vi "Memory.Pointer.Read.All.In Place.Safe (1D U8).vi"(8 "error in (no error)":errorcluster, 10 "buffer in":u8[](array[numeric]) format="%02x", 11 "Pointer in":refnum<class "Memory.Pointer.lvclass">) -> (0 "error out":errorcluster, 2 "buffer out":u8[](array[numeric]) format="%02x", 3 "Pointer out":refnum<class "Memory.Pointer.lvclass">)   [LabVIEW 2016, in "LabVIEW Memory Manager.lvlib" / "Memory.Pointer.lvclass"]
uses:
  Memory.Pointer.lvclass
  Memory.Pointer.lvclass/Memory.Pointer.ctl
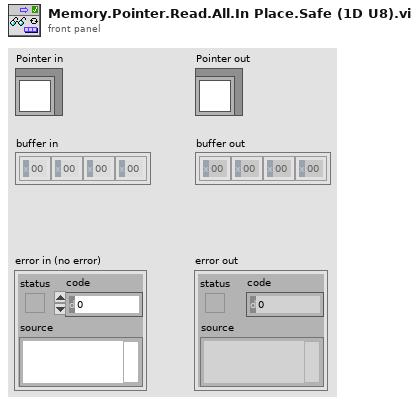
[diagram p1: front panel]
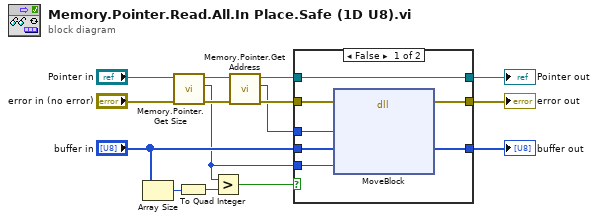
[diagram p0: block diagram]
diagram:
  n1 = Array Size(array="buffer in") -> (size(s)=w6:i32)
  n2 = call "Memory.Pointer.Get Size.vi"("error in (no error)"="error in (no error)", "Pointer in"="Pointer in") -> ("error out"=w15:errorcluster, "size"=w4:i64, "Pointer out"=w14:refnum<class "Memory.Pointer.lvclass">)  [unwired: 7 in]
  n3 = To Quad Integer(1:w6) -> (0:w5:i64)
  n4 = Greater?(x=w4, y=w5) -> (0:w1:bool)
  n5 = call "Memory.Pointer.Get Address.vi"("error in (no error)"=w15, "Pointer in"=w14) -> ("error out"=w13:errorcluster, "address"=w12:u64, "Pointer out"=w3:refnum<class "Memory.Pointer.lvclass">)  [unwired: 7 in]
  n6 = case shown="False" w1 {
    tunnel: w13 -> [w22 w24]
    tunnel: w12 -> [w21 _]
    tunnel: [w20 w23] -> w11
    tunnel: [w19 w24] -> w9
    tunnel: "buffer in" -> [w18 w23]
    tunnel: w4 -> [w17 _]
    tunnel: w3 -> [w16 w25]
    tunnel: [w16 w25] -> w2
    frame False {
      n7 = dll-call lib="LabVIEW" fn="MoveBlock"(error in=w22, "src pointer"=w21, "dst pointer"=w18, "size"=w17) -> (error out=w19:errorcluster, "dst pointer"=w20:u8[])  [unwired: 5 in, 1 out]
    }
    frame True {
      # "#TODO\nThrow error."
    }
  }
  "error out" <- w9
  "Pointer out" <- w2
  "buffer out" <- w11
